vi "Format Heading.vi"(0 "new heading":string, 1 "format string":string="### %s\\n", 2 "slashes to colons":bool, 7 "enable (T)":bool=TRUE, 11 "error in":errorcluster) -> (4 "string out":string, 15 "error out":errorcluster)   [LabVIEW 2019, in "MD Generator.lvlib"]
uses:
  MD Generator.lvlib
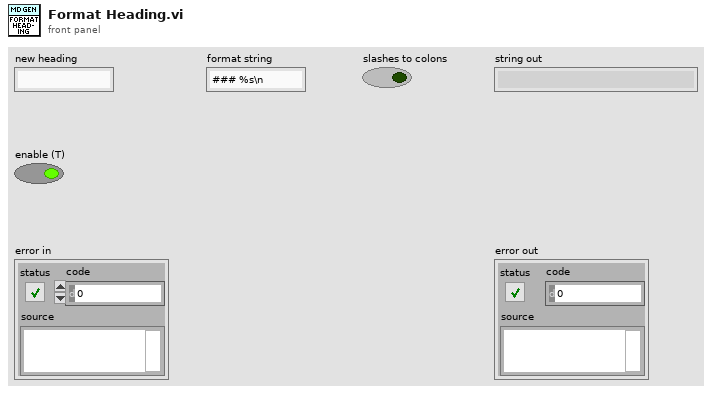
[diagram p1: front panel]
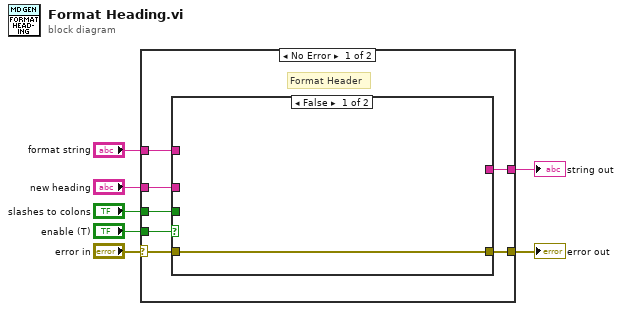
[diagram p0: block diagram]
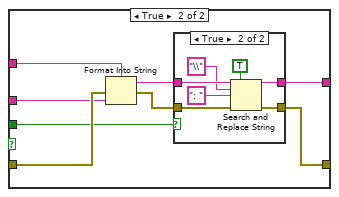
[diagram p2: hidden frame]
diagram:
  n1 = case shown="No Error" "error in" {
    selector: "error in" -> [w14 w33]
    tunnel: [w13 w33] -> w6
    tunnel: [w12 _] -> w5
    tunnel: "enable (T)" -> [w11 _]
    tunnel: "new heading" -> [w10 _]
    tunnel: "slashes to colons" -> [w9 _]
    tunnel: "format string" -> [w8 _]
    frame No Error {
      # "Format Header"
      n2 = case shown="False" w11 {
        tunnel: [_ w20] -> w12
        tunnel: w10 -> [_ w22]
        tunnel: [w15 w19] -> w13
        tunnel: w14 -> [w15 w23]
        tunnel: w9 -> [_ w17]
        tunnel: w8 -> [_ w16]
        frame False {
        }
        frame True {
          n3 = Format Into String(format string=w16, error in=w23, w22) -> (resulting string=w21:string, error out=w18:errorcluster)  [unwired: 1 in]
          n4 = case shown="True" w17 {
            tunnel: w21 -> [w25 w32]
            tunnel: [w25 w31] -> w20
            tunnel: [w24 w29] -> w19
            tunnel: w18 -> [w24 w27]
            frame False {
            }
            frame True {
              n5 = Search and Replace String(replace all?=TRUE ("replace all? (F)"), input string=w32, search string="\\", replace string=": " ("replace string (\"\")"), error in=w27) -> (result string=w31:string, error out=w29:errorcluster)  [unwired: 3 in, 2 out]
            }
          }
        }
      }
    }
    frame Error {
    }
  }
  "error out" <- w6
  "string out" <- w5
